vi "saveImages.vi"(8 "error in (no error)":errorcluster, 10 "Array":path[](array[path]), 11 "Pixelfly in":refnum<class "Pixelfly.lvclass">) -> (0 "error out":errorcluster, 3 "Pixelfly out":refnum<class "Pixelfly.lvclass">)   [LabVIEW 2009, in "Hardware.lvlib" / "Channels.lvlib" / "Pixelfly.lvclass"]
uses:
  Pixelfly.lvclass
  Camera.lvclass
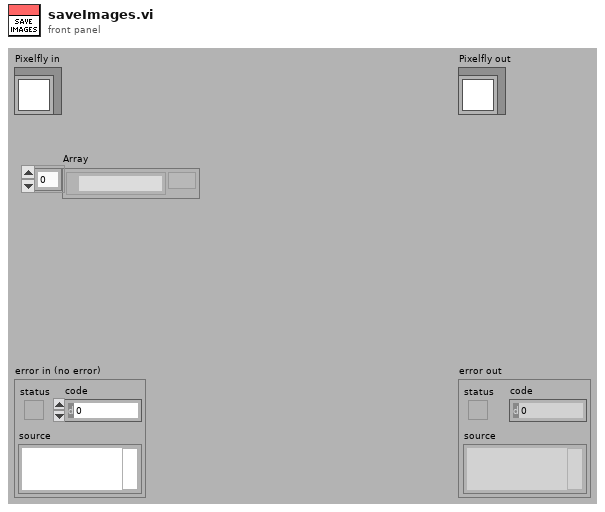
[diagram p1: front panel]
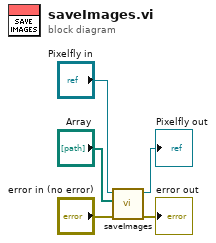
[diagram p0: block diagram]
diagram:
  n1 = call-parent "saveImages.vi"("error in (no error)"="error in (no error)", "Array"="Array", "Camera in"="Pixelfly in") -> ("error out"=→"error out":errorcluster, "Camera out"=→"Pixelfly out":refnum<class "Pixelfly.lvclass">)  [unwired: 7 in]
